vi "Line Extraction.vi"(8 "error in (no error)":errorcluster, 9 "element":cluster{i32[], dbl[]}, 10 "XY Array":T1[](array[typedef])) -> (0 "error out":errorcluster, 1 "Strength":dbl, 2 "Distance from Wall":dbl, 3 "Angle":dbl)   [LabVIEW 2017]
uses:
  040-typeDefs/LidarPoint.ctl
panel:
  out "XY Graph":cluster{i32[], dbl[]}[](graph)
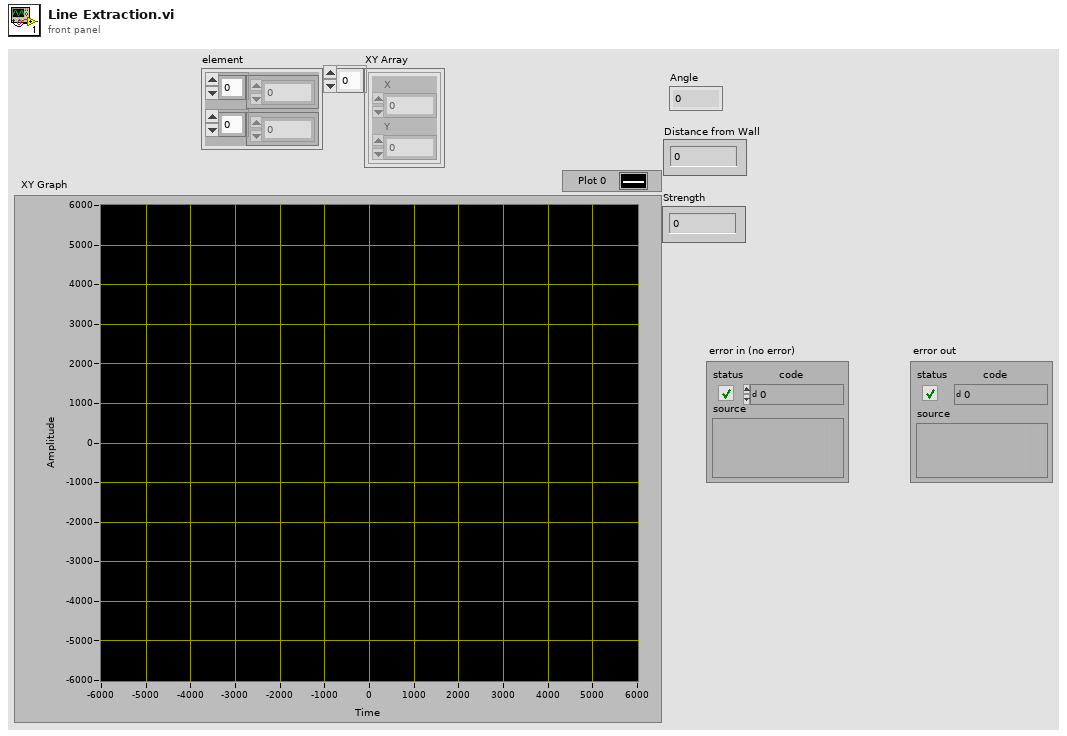
[diagram p1: front panel]
types:
  T1 = typedef "LidarPoint.ctl" = cluster{"X":dbl, "Y":dbl}
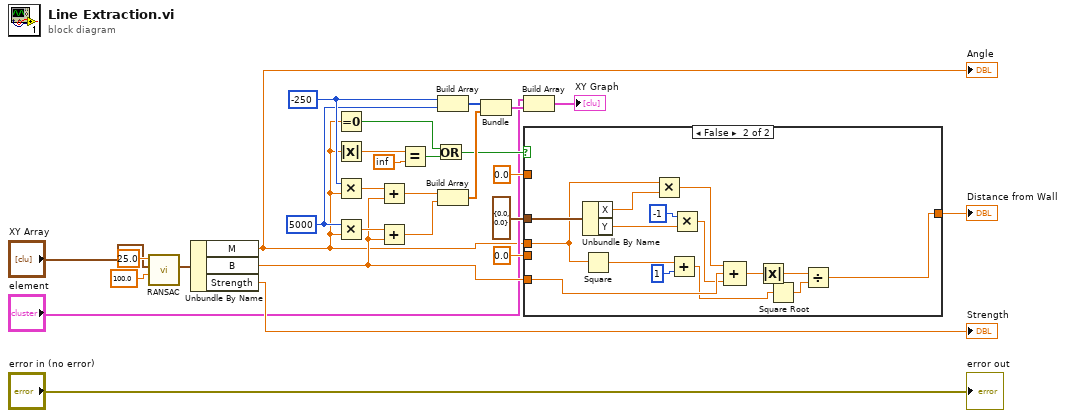
[diagram p0: block diagram]
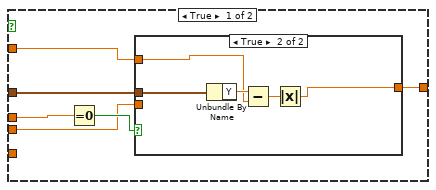
[diagram p2: hidden frame]
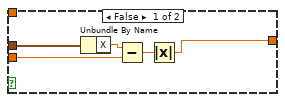
[diagram p3: hidden frame]
diagram:
  w23 = 5000
  w24 = -250
  n1 = call "RANSAC.vi"("Checks"=100.0, "XY Array"="XY Array", "Tolerance"=25.0) -> ("Best Line"=w27:cluster{"M":dbl, "B":dbl, "Strength":dbl})  [unwired: 8 in]
  n2 = Unbundle By Name(w27) -> ("M"=w1:dbl, "B"=w9:dbl, "Strength"=→"Strength":dbl)
  "Angle" <- w1
  n3 = Equal To 0?(x=w1) -> (x = 0?=w12:bool)
  n4 = Absolute Value(x=w1) -> (abs(x)=w14:dbl)
  n5 = Multiply(x=w24, y=w1) -> (x*y=w26:dbl)
  n6 = Multiply(x=w23, y=w1) -> (x*y=w25:dbl)
  n7 = Add(x=w26, y=w9) -> (x+y=w21:dbl)
  n8 = Add(x=w25, y=w9) -> (x+y=w22:dbl)
  n9 = Equal?(x=w14, y=inf) -> (x = y?=w11:bool)
  n10 = Or(x=w12, y=w11) -> (x .or. y?=w10:bool)
  n11 = Build Array(w24, w23) -> (w18:i32[])
  n12 = Build Array(w21, w22) -> (w17:dbl[])
  n13 = Bundle(w18, w17) -> (w20:cluster{i32[], dbl[]})  [unwired: 1 in]
  n14 = Build Array("element", w20) -> (→"XY Graph":cluster{i32[], dbl[]}[])
  n15 = case shown="False" w10 {
    tunnel: w9 -> [_ w54]
    tunnel: T1 {"X"=0.0, "Y"=0.0} ("XY") -> [w32 w59]
    tunnel: [w30 w45] -> w6
    tunnel: 0.0 ("X") -> [w31 _]
    tunnel: 0.0 ("Y") -> [w29 _]
    tunnel: w1 -> [w33 w49]
    frame True {
      n16 = Equal To 0?(x=w33) -> (x = 0?=w34:bool)
      n17 = case shown="True" w34 {
        tunnel: w32 -> [w39 w44]
        tunnel: w31 -> [w37 _]
        tunnel: [w35 w40] -> w30
        tunnel: w29 -> [_ w41]
        frame False {
          n18 = Unbundle By Name(w39) -> ("X"=w38:dbl)
          n19 = Subtract(x=w38, y=w37) -> (x-y=w36:dbl)
          n20 = Absolute Value(x=w36) -> (abs(x)=w35:dbl)
        }
        frame True {
          n21 = Unbundle By Name(w44) -> ("Y"=w43:dbl)
          n22 = Subtract(x=w43, y=w41) -> (x-y=w42:dbl)
          n23 = Absolute Value(x=w42) -> (abs(x)=w40:dbl)
        }
      }
    }
    frame False {
      n24 = Unbundle By Name(w59) -> ("X"=w56:dbl, "Y"=w57:dbl)
      n25 = Square(x=w49) -> (x^2=w51:dbl)
      n26 = Multiply(x=w49, y=w56) -> (x*y=w55:dbl)
      n27 = Add(x=w51, y=1) -> (x+y=w46:dbl)
      n28 = Multiply(x=-1, y=w57) -> (x*y=w53:dbl)
      n29 = Compound Arithmetic op=ADD(w55, w54, w53) -> (w52:dbl)
      n30 = Absolute Value(x=w52) -> (abs(x)=w48:dbl)
      n31 = Square Root(x=w46) -> (sqrt(x)=w47:dbl)
      n32 = Divide(x=w48, y=w47) -> (x/y=w45:dbl)
    }
  }
  "Distance from Wall" <- w6
  "error out" <- "error in (no error)"
